vi "Read Pressure Unit.vi"(7 "Channel (0: Channel A)":u16(ring) items=["Channel A", "Channel B"], 8 "error in (no error)":errorcluster, 11 "BH Druck PACE Series in":refnum<class "BH Druck PACE Series.lvclass">) -> (0 "error out":errorcluster, 1 "Unit Convert":dbl, 2 "Selected Unit":string="mbar", 3 "BH Druck PACE Series out":refnum<class "BH Druck PACE Series.lvclass">)   [LabVIEW 2022 SP3, in "BH Druck PACE Series.lvclass"]
uses:
  BH Druck PACE Series.lvclass
  BH Druck PACE Series.lvclass/BH Druck PACE Series.ctl
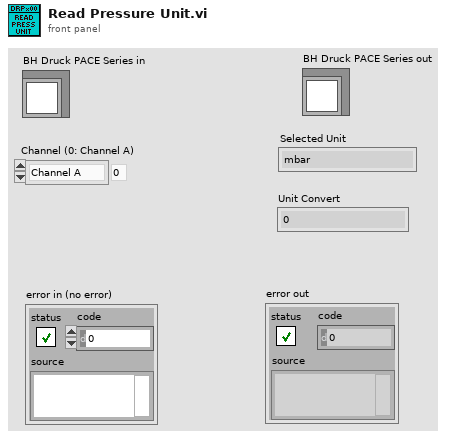
[diagram p1: front panel]
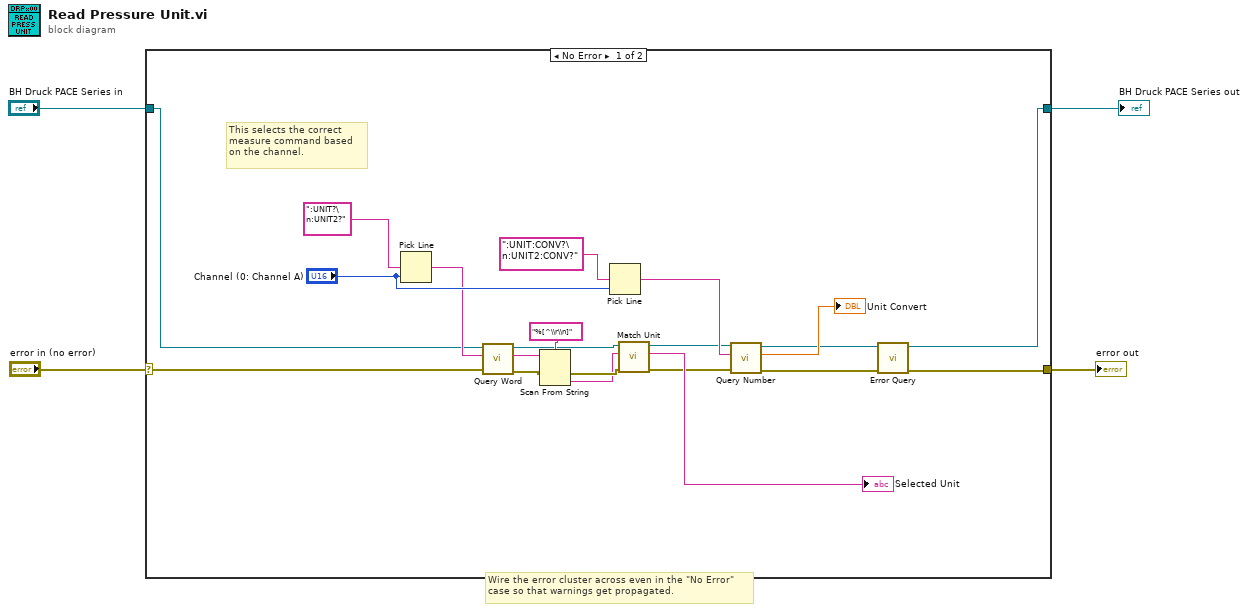
[diagram p0: block diagram]
diagram:
  # "Wire the error cluster across even in the \"No Error\"\ncase so that warnings get propagated."
  n1 = case shown="No Error" "error in (no error)" {
    selector: "error in (no error)" -> [w14 w27]
    tunnel: [w13 w27] -> w3
    tunnel: [w5 w26] -> w1
    tunnel: "BH Druck PACE Series in" -> [w12 w26]
    frame No Error {
      # "This selects the correct\nmeasure command based\non the channel."
      n2 = Pick Line(multi-line string=":UNIT?\n:UNIT2?", line index="Channel (0: Channel A)") -> (output string=w19:string)  [unwired: 1 in]
      n3 = call-dynamic "Query Word.vi"("error in (no error)"=w14, "Query String"=w19, "BH Druck PACE Series in"=w12) -> ("error out"=w11:errorcluster, "String Result"=w25:string, "BH Druck PACE Series out"=w8:refnum<class "BH Druck PACE Series.lvclass">)  [unwired: 6 in]
      n4 = Scan From String(format string="%[^\\r\\n]", input string=w25, error in=w11) -> (error out=w10:errorcluster, output 1=w9:string)  [unwired: 2 in, 2 out]
      n5 = Pick Line(multi-line string=":UNIT:CONV?\n:UNIT2:CONV?", line index="Channel (0: Channel A)") -> (output string=w21:string)  [unwired: 1 in]
      n6 = call-dynamic "Match Unit.vi"("error in (no error)"=w10, "Unit Read"=w9, "BH Druck PACE Series in"=w8) -> ("error out"=w15:errorcluster, "Unit Display"=→"Selected Unit":string, "BH Druck PACE Series out"=w7:refnum<class "BH Druck PACE Series.lvclass">)  [unwired: 6 in]
      n7 = call-dynamic "Query Number.vi"("error in (no error)"=w15, "Query String"=w21, "BH Druck PACE Series in"=w7) -> ("error out"=w20:errorcluster, "Numeric Result"=→"Unit Convert":dbl, "BH Druck PACE Series out"=w6:refnum<class "BH Druck PACE Series.lvclass">)  [unwired: 6 in]
      n8 = call-dynamic "Error Query.vi"("error in (no error)"=w20, "BH Druck PACE Series in"=w6) -> ("error out"=w13:errorcluster, "BH Druck PACE Series out"=w5:refnum<class "BH Druck PACE Series.lvclass">)  [unwired: 8 in]
    }
    frame Error {
    }
  }
  "error out" <- w3
  "BH Druck PACE Series out" <- w1
